vi "set properties.vi"   [LabVIEW 2020, in "type.lvclass"]
uses:
  type.lvclass
  type.lvclass/type.ctl
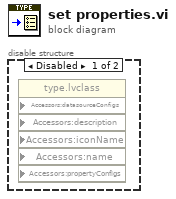
[diagram p0: block diagram]
diagram:
  n1 = disable-structure shown="Disabled" {
    frame Disabled {
      n2 = property class="type.lvclass" props=["Accessors:datasourceConfigs", "Accessors:description", "Accessors:iconName", "Accessors:name", "Accessors:propertyConfigs"]() -> ()  [unwired: 7 in, 2 out]
    }
    frame Enabled {
    }
  }
